vi "LIN EX Decode List File.vi"(0 "pFileName":string, 1 "ReadDataListLen":i8, 2 "CheckTypeListLen":i8, 5 "CheckType":i8, 7 "BaudRate":i32, 9 "pReadDataList":string, 11 "error in (no error)":errorcluster, 12 "pCheckTypeList":string) -> (4 "pFileName out":string, 6 "function return":i32, 10 "pReadDataList out":string, 14 "pCheckTypeList out":string, 15 "error out":errorcluster)   [LabVIEW 2010, in "usb2lin_ex.lvlib"]
doc: "int WINAPI LIN_EX_DecodeListFile(char *pFileName,char CheckType,int BaudRate,char *pReadDataList,char ReadDataListLen,char *pCheckTypeList,char CheckTypeListLen);"
uses:
  usb2lin_ex.lvlib
  USB2XXX.dll
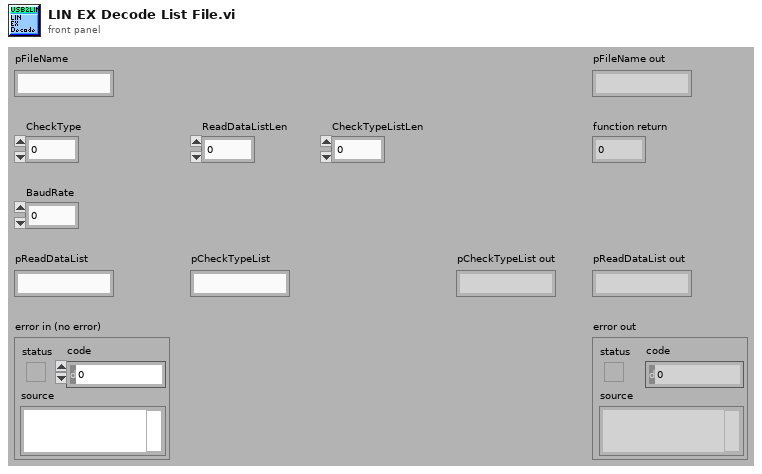
[diagram p1: front panel]
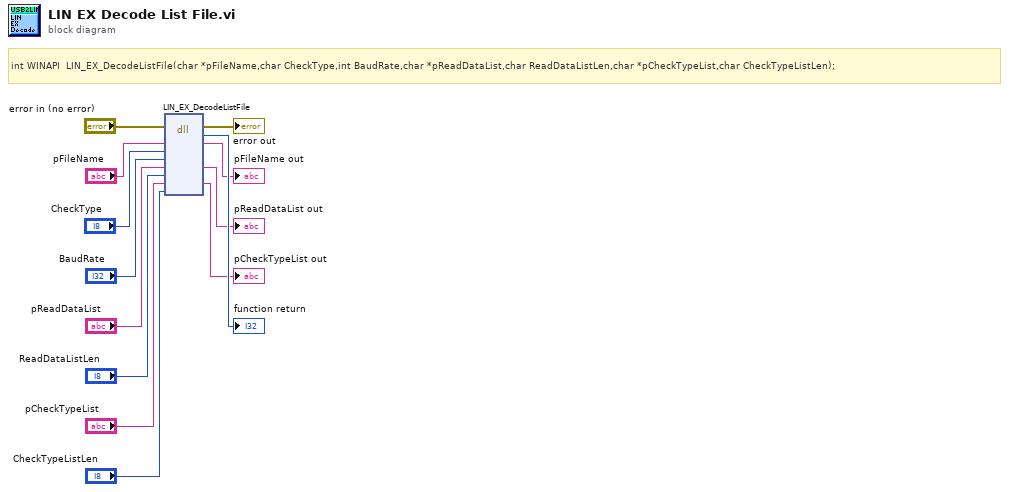
[diagram p0: block diagram]
diagram:
  # "int WINAPI  LIN_EX_DecodeListFile(char *pFileName,char CheckType,int BaudRate,char *pReadDataList,char ReadDataListLen,char *pCheckTypeList,char CheckTypeListLen);"
  n1 = dll-call lib="E:/OtherWork/STM32/USB2XXX_Example/sdk/api/Labview/USB2XXX.*" fn="LIN_EX_DecodeListFile"(error in="error in (no error)", "pFileName"="pFileName", "CheckType"="CheckType", "BaudRate"="BaudRate", "pReadDataList"="pReadDataList", "ReadDataListLen"="ReadDataListLen", "pCheckTypeList"="pCheckTypeList", "CheckTypeListLen"="CheckTypeListLen") -> (error out=→"error out":errorcluster, →"function return":i32, "pFileName"=→"pFileName out":string, "pReadDataList"=→"pReadDataList out":string, "pCheckTypeList"=→"pCheckTypeList out":string)  [unwired: 6 in, 1 out]
